vi "maj1.vi"() -> ()   [LabVIEW 2023]
panel:
  out "Czy istnieja pierwiastki?":string
  out "Pierwiastek 2":dbl
  out "Pierwiastek 1":dbl
  in  "c":dbl
  in  "b":dbl
  in  "a":dbl
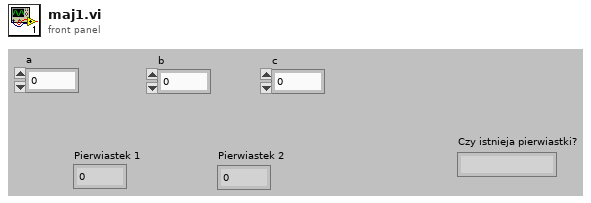
[diagram p1: front panel]
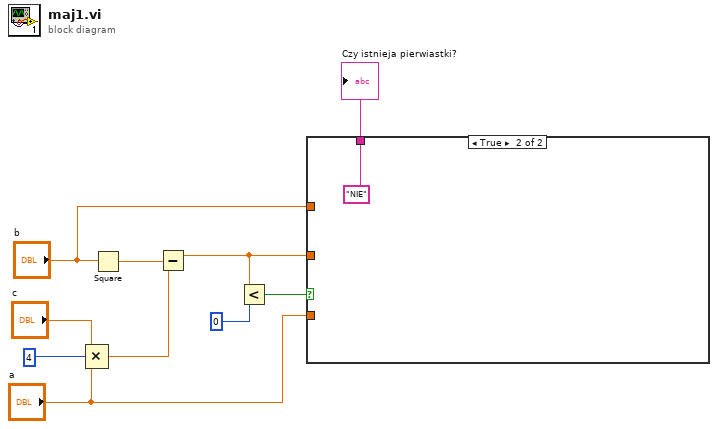
[diagram p0: block diagram]
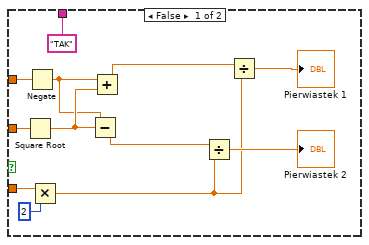
[diagram p2: hidden frame]
diagram:
  n1 = Compound Arithmetic op=MULTIPLY("a", 4, "c") -> (w8:dbl)
  n2 = Square(x="b") -> (x^2=w7:dbl)
  n3 = Subtract(x=w7, y=w8) -> (x-y=w3:dbl)
  n4 = Less?(x=w3, y=0) -> (x < y?=w5:bool)
  n5 = case shown="True" w5 {
    tunnel: ["TAK" "NIE"] -> w4
    tunnel: w3 -> [w21 _]
    tunnel: "b" -> [w20 _]
    tunnel: "a" -> [w18 _]
    frame False {
      n6 = Square Root(x=w21) -> (sqrt(x)=w17:dbl)
      n7 = Negate(x=w20) -> (-x=w16:dbl)
      n8 = Multiply(x=w18, y=2) -> (x*y=w11:dbl)
      n9 = Subtract(x=w16, y=w17) -> (x-y=w12:dbl)
      n10 = Add(x=w16, y=w17) -> (x+y=w13:dbl)
      n11 = Divide(x=w12, y=w11) -> (x/y=→"Pierwiastek 2":dbl)
      n12 = Divide(x=w13, y=w11) -> (x/y=→"Pierwiastek 1":dbl)
    }
    frame True {
    }
  }
  "Czy istnieja pierwiastki?" <- w4
